vi "Test Queue Operations.vi"() -> ()   [LabVIEW 2013]
uses:
  <vilib>/addons/_JKI Toolkits/Caraya/classes/Assert/Assert True.vi
  Circular Buffers/ByteFIFO/ByteFIFO.lvclass
  Circular Buffers/VariantBuffer/VariantBuffer.lvclass
  <vilib>/addons/_JKI Toolkits/Caraya/classes/Test/Test.lvclass
  <vilib>/addons/_JKI Toolkits/Caraya/classes/Assert/Assert.lvclass
panel:
  out "15 element overflow":u8[](array[numeric]) format="%02x"
  out "index2 byte":u8 format="%02x"
  out "flushed":u8[](array[numeric]) format="%02x"
  out "5 element overflow":u8[](array[numeric]) format="%02x"
  out "10 more element overflow":u8[](array[numeric]) format="%02x"
  out "last 5 elements":u8[](array[numeric]) format="%02x"
  out "dequeued":u8[](array[numeric]) format="%02x"
  out "overflow":u8[](array[numeric]) format="%02x"
  out "error out":errorcluster
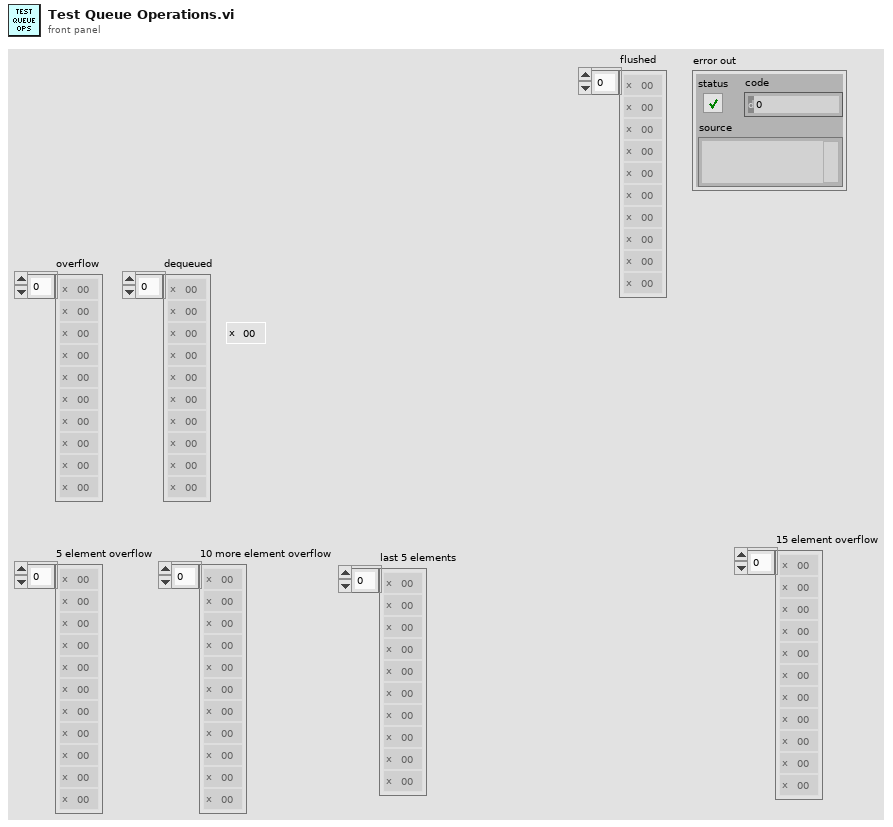
[diagram p1: front panel]
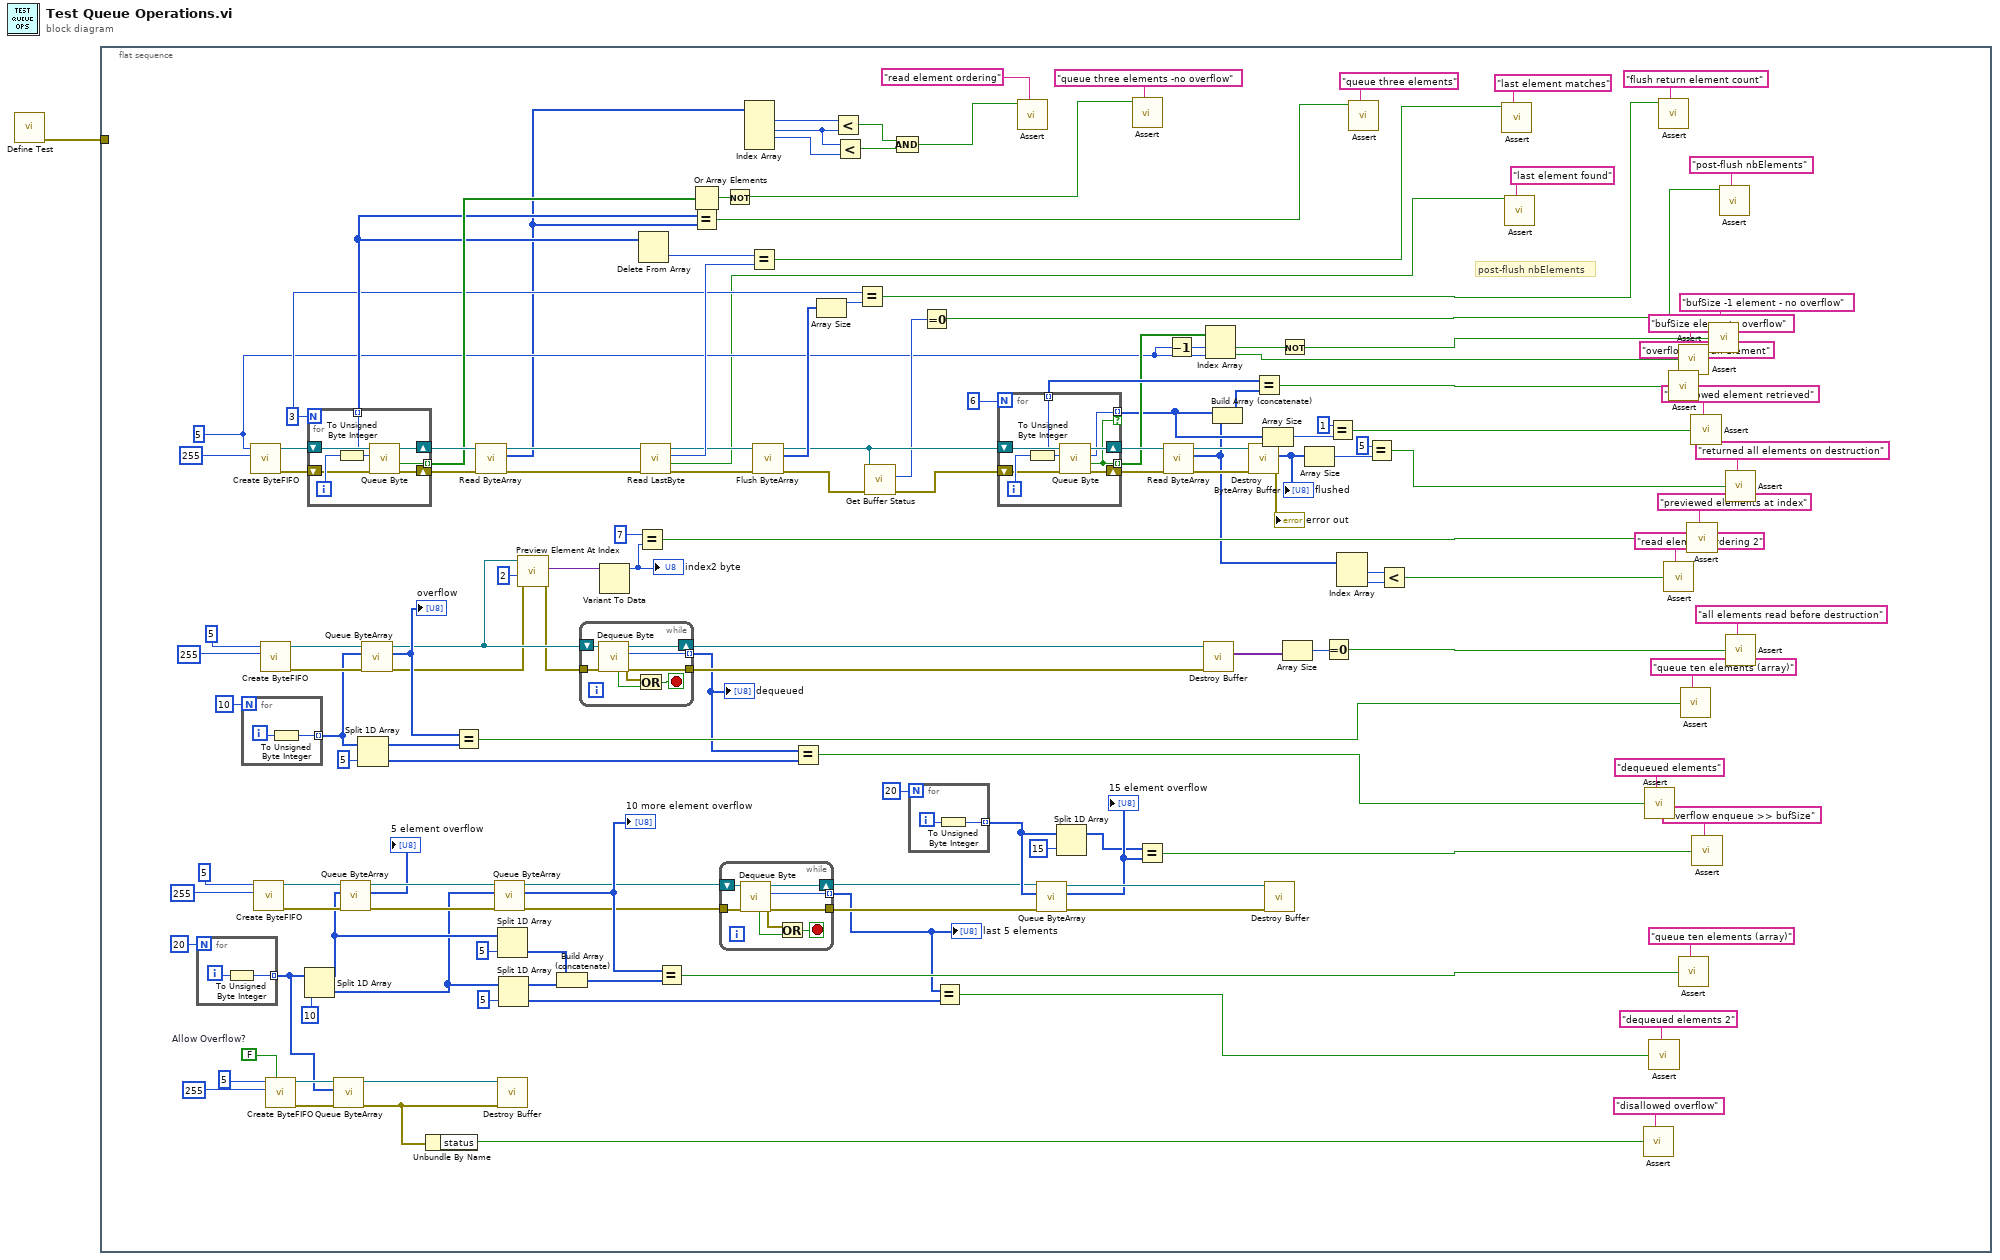
[diagram p0: block diagram]
diagram:
  n1 = call <vilib>:"Define Test.vi"() -> ("error out"=w1:errorcluster)  [unwired: 10 in, 1 out]
  n2 = flat-sequence {
    tunnel: w1 -> [_]
    frame #0 {
      w48 = FALSE  # Allow Overflow?
      w138 = 3
      w124 = 5 ("bufSize")
      # "post-flush nbElements"
      n3 = for {
        N: 20 -> [_]
        tunnel: [w154] -> w45 mode=indexing
        i -> [w155]
        n4 = To Unsigned Byte Integer(number=w155) -> (unsigned 8bit integer=w154:u8)
      }
      n5 = for {
        N: 10 -> [_]
        tunnel: [w163] -> w101 mode=indexing
        i -> [w164]
        n6 = To Unsigned Byte Integer(number=w164) -> (unsigned 8bit integer=w163:u8)
      }
      n7 = call "Create ByteFIFO.vi"("default value"=u8 255, "bufSize"=w124) -> ("error out"=w136:errorcluster, "Buffer"=w150:refnum<data-value>)  [unwired: 8 in]
      n8 = call "Create ByteFIFO.vi"("default value"=u8 255, "bufSize"=5) -> ("error out"=w84:errorcluster, "Buffer"=w82:refnum<data-value>)  [unwired: 8 in]
      n9 = call "Create ByteFIFO.vi"("default value"=u8 255, "bufSize"=5) -> ("error out"=w109:errorcluster, "Buffer"=w110:refnum<data-value>)  [unwired: 8 in]
      n10 = call "Create ByteFIFO.vi"("Allow Overflow? (T)"=w48, "default value"=u8 255, "bufSize"=5) -> ("error out"=w46:errorcluster, "Buffer"=w47:refnum<data-value>)  [unwired: 7 in]
      n11 = Split 1D Array(array=w45, index=10) -> (first subarray=w74:u8[], second subarray=w72:u8[])
      n12 = for {
        N: w138 -> [_]
        shift-right: [w184] -> w149
        shift-left: w150 -> [w186]
        tunnel: [w183] -> w144 mode=indexing
        tunnel: [w182] -> w147 mode=indexing
        shift-right: [w180] -> w135
        shift-left: w136 -> [w181]
        i -> [w185]
        n13 = To Unsigned Byte Integer(number=w185) -> (unsigned 8bit integer=w183:u8)
        n14 = call "Queue Byte.vi"("error in"=w181, "byte"=w183, "Buffer"=w186) -> ("error out"=w180:errorcluster, "overflowed?"=w182:bool, "Buffer"=w184:refnum<data-value>)  [unwired: 5 in, 1 out]
      }
      n15 = call "Queue ByteArray.vi"("error in"=w46, "bytes"=w45, "Buffer"=w47) -> ("error out"=w43:errorcluster, "Buffer"=w44:refnum<data-value>)  [unwired: 6 in, 1 out]
      n16 = call "Queue ByteArray.vi"("error in"=w84, "bytes"=w74, "Buffer"=w82) -> ("error out"=w83:errorcluster, "overflow"=→"5 element overflow":u8[], "Buffer"=w81:refnum<data-value>)  [unwired: 6 in]
      n17 = Split 1D Array(array=w101, index=5) -> (first subarray=w95:u8[], second subarray=w94:u8[])
      n18 = call "Queue ByteArray.vi"("error in"=w109, "bytes"=w101, "Buffer"=w110) -> ("error out"=w69:errorcluster, "overflow"=w102:u8[], "Buffer"=w70:refnum<data-value>)  [unwired: 6 in]
      "overflow" <- w102
      n19 = Unbundle By Name(w43) -> ("status"=w42:bool)
      n20 = Equal?(x=w102, y=w95) -> (x = y?=w99:bool)
      n21 = call "Read ByteArray.vi"("error in"=w135, "Buffer"=w149) -> ("error out"=w134:errorcluster, "bytes"=w31:u8[], "Buffer"=w148:refnum<data-value>)  [unwired: 7 in]
      n22 = call "Queue ByteArray.vi"("error in"=w83, "bytes"=w72, "Buffer"=w81) -> ("error out"=w87:errorcluster, "overflow"=w88:u8[], "Buffer"=w50:refnum<data-value>)  [unwired: 6 in]
      "10 more element overflow" <- w88
      n23 = Split 1D Array(array=w74, index=5) -> (second subarray=w73:u8[])  [unwired: 1 out]
      n24 = call "Destroy Buffer.vi"("error in"=w43, "Buffer"=w44) -> ()  [unwired: 8 in, 2 out]
      n25 = Split 1D Array(array=w72, index=5) -> (first subarray=w77:u8[], second subarray=w91:u8[])
      n26 = call "Preview Element At Index.vi"("error in"=w69, "index"=2 ("index (-1: last)"), "Buffer in"=w70) -> ("error out"=w68:errorcluster, "element"=w66:variant)  [unwired: 5 in, 2 out]
      n27 = Build Array (concatenate)(w73, w77) -> (w76:u8[])
      n28 = while {
        tunnel: w68 -> [w169]
        tunnel: [w167] -> w106
        tunnel: [w168] -> w41 mode=indexing
        shift-right: [w170] -> w107
        shift-left: w70 -> [w171]
        stop <- w166 stop-if-true
        n29 = call "Dequeue Byte.vi"("error in"=w169, "Buffer"=w171) -> ("error out"=w167:errorcluster, "byte"=w168:u8, "Buffer"=w170:refnum<data-value>, "buffer empty?"=w165:bool)  [unwired: 5 in, 1 out]
        n30 = Or(x=w167, y=w165) -> (x .or. y?=w166:bool)
      }
      "dequeued" <- w41
      n31 = Variant To Data(Variant=w66) -> (data=w65:u8)  [unwired: 2 in, 1 out]
      "index2 byte" <- w65
      n32 = Equal?(x=u8 7, y=w65) -> (x = y?=w63:bool)
      n33 = Delete From Array(array=w144) -> (deleted portion=w143:u8)  [unwired: 2 in, 1 out]
      n34 = call "Read LastByte.vi"("error in"=w134, "Buffer"=w148) -> ("error out"=w133:errorcluster, "found"=w21:bool, "byte"=w145:u8, "Buffer"=w141:refnum<data-value>)  [unwired: 6 in]
      n35 = Equal?(x=w88, y=w76) -> (x = y?=w90:bool)
      n36 = Or Array Elements(Boolean array=w147) -> (logical OR=w146:bool)
      n37 = Equal?(x=w144, y=w31) -> (x = y?=w25:bool)
      n38 = while {
        tunnel: w87 -> [w161]
        tunnel: [w157] -> w60
        tunnel: [w160] -> w51 mode=indexing
        shift-right: [w159] -> w49
        shift-left: w50 -> [w162]
        stop <- w158 stop-if-true
        n39 = call "Dequeue Byte.vi"("error in"=w161, "Buffer"=w162) -> ("error out"=w157:errorcluster, "byte"=w160:u8, "Buffer"=w159:refnum<data-value>, "buffer empty?"=w156:bool)  [unwired: 5 in, 1 out]
        n40 = Or(x=w157, y=w156) -> (x .or. y?=w158:bool)
      }
      "last 5 elements" <- w51
      n41 = Not(x=w146) -> (.not. x?=w28:bool)
      n42 = Index Array(array=w31) -> (element #1=w36:u8, element #2=w35:u8, element #3=w34:u8)  [unwired: 4 in, 1 out]
      n43 = Equal?(x=w143, y=w145) -> (x = y?=w23:bool)
      n44 = call "Flush ByteArray.vi"("error in"=w133, "Buffer"=w141) -> ("error out"=w132:errorcluster, "bytes"=w140:u8[], "Buffer"=w137:refnum<data-value>)  [unwired: 7 in]
      n45 = Equal?(x=w41, y=w94) -> (x = y?=w93:bool)
      n46 = Array Size(array=w140) -> (size(s)=w139:i32)
      n47 = Less?(x=w36, y=w35) -> (x < y?=w32:bool)
      n48 = Less?(x=w35, y=w34) -> (x < y?=w33:bool)
      n49 = Equal?(x=w138, y=w139) -> (x = y?=w19:bool)
      n50 = call "Get Buffer Status.vi"("error in"=w132, "Buffer in"=w137) -> ("error out"=w131:errorcluster, "nbElements"=w130:i32)  [unwired: 5 in, 3 out]
      n51 = Compound Arithmetic op=AND(w32, w33) -> (w30:bool)
      n52 = for {
        N: 20 -> [_]
        tunnel: [w152] -> w57 mode=indexing
        i -> [w153]
        n53 = To Unsigned Byte Integer(number=w153) -> (unsigned 8bit integer=w152:u8)
      }
      n54 = Equal To 0?(x=w130) -> (x = 0?=w18:bool)
      n55 = Equal?(x=w51, y=w91) -> (x = y?=w92:bool)
      n56 = for {
        N: 6 -> [_]
        shift-right: [w177] -> w127
        shift-left: w137 -> [w179]
        tunnel: [w174] -> w129 mode=indexing
        tunnel: [w172] -> w126 mode=indexing
        shift-right: [w175] -> w128
        shift-left: w131 -> [w176]
        tunnel: [w173] -> w118 mode=indexing if=w172
        i -> [w178]
        n57 = To Unsigned Byte Integer(number=w178) -> (unsigned 8bit integer=w174:u8)
        n58 = call "Queue Byte.vi"("error in"=w176, "byte"=w174, "Buffer"=w179) -> ("error out"=w175:errorcluster, "overflowed?"=w172:bool, "overflow"=w173:u8, "Buffer"=w177:refnum<data-value>)  [unwired: 5 in]
      }
      n59 = call-poly <vilib>:"Assert.vi"("Label"="read element ordering", "True?"=w30) -> ()  [unwired: 8 in, 2 out]
      n60 = call "Queue ByteArray.vi"("error in"=w60, "bytes"=w57, "Buffer"=w49) -> ("error out"=w61:errorcluster, "overflow"=w56:u8[], "Buffer"=w62:refnum<data-value>)  [unwired: 6 in]
      "15 element overflow" <- w56
      n61 = Split 1D Array(array=w57, index=15) -> (first subarray=w54:u8[])  [unwired: 1 out]
      n62 = call-poly <vilib>:"Assert.vi"("Label"="queue three elements -no overflow", "True?"=w28) -> ()  [unwired: 8 in, 2 out]
      n63 = Equal?(x=w54, y=w56) -> (x = y?=w55:bool)
      n64 = call "Read ByteArray.vi"("error in"=w128, "Buffer"=w127) -> ("error out"=w113:errorcluster, "bytes"=w38:u8[], "Buffer"=w114:refnum<data-value>)  [unwired: 7 in]
      n65 = Decrement(x=w124) -> (x-1=w125:i32)
      n66 = call "Destroy Buffer.vi"("error in"=w106, "Buffer"=w107) -> ("elements"=w98:variant[])  [unwired: 8 in, 1 out]
      n67 = Index Array(array=w126, index #1=w125, index #2=w124) -> (element #1=w123:bool, element #2=w122:bool)
      n68 = Build Array (concatenate)(w118, w38) -> (w120:u8[])
      n69 = call "Destroy ByteArray Buffer.vi"("error in"=w113, "Buffer"=w114) -> ("error out"=→"error out":errorcluster, "bytes"=w71:u8[])  [unwired: 8 in]
      "flushed" <- w71
      n70 = Equal?(x=w129, y=w120) -> (x = y?=w121:bool)
      n71 = Array Size(array=w118) -> (size(s)=w119:i32)
      n72 = call "Destroy Buffer.vi"("error in"=w61, "Buffer"=w62) -> ()  [unwired: 8 in, 2 out]
      n73 = Not(x=w123) -> (.not. x?=w115:bool)
      n74 = Array Size(array=w98) -> (size(s)=w97:i32)
      n75 = Array Size(array=w71) -> (size(s)=w104:i32)
      n76 = Equal To 0?(x=w97) -> (x = 0?=w96:bool)
      n77 = Equal?(x=1, y=w119) -> (x = y?=w116:bool)
      n78 = Index Array(array=w38) -> (element #1=w39:u8, element #2=w40:u8)  [unwired: 2 in]
      n79 = call-poly <vilib>:"Assert.vi"("Label"="queue three elements", "True?"=w25) -> ()  [unwired: 8 in, 2 out]
      n80 = Equal?(x=5, y=w104) -> (x = y?=w103:bool)
      n81 = Less?(x=w39, y=w40) -> (x < y?=w37:bool)
      n82 = call-poly <vilib>:"Assert.vi"("Label"="last element matches", "True?"=w23) -> ()  [unwired: 8 in, 2 out]
      n83 = call-poly <vilib>:"Assert.vi"("Label"="last element found", "True?"=w21) -> ()  [unwired: 8 in, 2 out]
      n84 = call-poly <vilib>:"Assert.vi"("Label"="disallowed overflow", "True?"=w42) -> ()  [unwired: 8 in, 2 out]
      n85 = call-poly <vilib>:"Assert.vi"("Label"="dequeued elements", "True?"=w93) -> ()  [unwired: 8 in, 2 out]
      n86 = call-poly <vilib>:"Assert.vi"("Label"="dequeued elements 2", "True?"=w92) -> ()  [unwired: 8 in, 2 out]
      n87 = call-poly <vilib>:"Assert.vi"("Label"="flush return element count", "True?"=w19) -> ()  [unwired: 8 in, 2 out]
      n88 = call-poly <vilib>:"Assert.vi"("Label"="read element ordering 2", "True?"=w37) -> ()  [unwired: 8 in, 2 out]
      n89 = call-poly <vilib>:"Assert.vi"("Label"="overflow loss an element", "True?"=w121) -> ()  [unwired: 8 in, 2 out]
      n90 = call-poly <vilib>:"Assert.vi"("Label"="bufSize element - overflow", "True?"=w122) -> ()  [unwired: 8 in, 2 out]
      n91 = call-poly <vilib>:"Assert.vi"("Label"="queue ten elements (array)", "True?"=w90) -> ()  [unwired: 8 in, 2 out]
      n92 = call-poly <vilib>:"Assert.vi"("Label"="queue ten elements (array)", "True?"=w99) -> ()  [unwired: 8 in, 2 out]
      n93 = call-poly <vilib>:"Assert.vi"("Label"="previewed elements at index", "True?"=w63) -> ()  [unwired: 8 in, 2 out]
      n94 = call-poly <vilib>:"Assert.vi"("Label"="overflowed element retrieved", "True?"=w116) -> ()  [unwired: 8 in, 2 out]
      n95 = call-poly <vilib>:"Assert.vi"("Label"="overflow enqueue >> bufSize", "True?"=w55) -> ()  [unwired: 8 in, 2 out]
      n96 = call-poly <vilib>:"Assert.vi"("Label"="bufSize -1 element - no overflow", "True?"=w115) -> ()  [unwired: 8 in, 2 out]
      n97 = call-poly <vilib>:"Assert.vi"("Label"="post-flush nbElements", "True?"=w18) -> ()  [unwired: 8 in, 2 out]
      n98 = call-poly <vilib>:"Assert.vi"("Label"="returned all elements on destruction", "True?"=w103) -> ()  [unwired: 8 in, 2 out]
      n99 = call-poly <vilib>:"Assert.vi"("Label"="all elements read before destruction", "True?"=w96) -> ()  [unwired: 8 in, 2 out]
    }
  }
